vi "Annotation Holder.vi"(0 "Index":i32, 1 "Action":T2, 5 "Start time":timestamp, 7 "Annotation in":T1, 9 "End Time":timestamp, 11 "error in (no error)":errorcluster, 12 "Array of annotations in":T1[](array[typedef])) -> (4 "Index & Size Out":i32, 6 "Array of Indexes":i32[](array[numeric]), 8 "Annotation out":T1, 10 "Array Of annotations":T1[](array[typedef]), 15 "error out":errorcluster)   [LabVIEW 2011]
uses:
  Actin Annotatino Holder.ctl
  Annotation Message.ctl
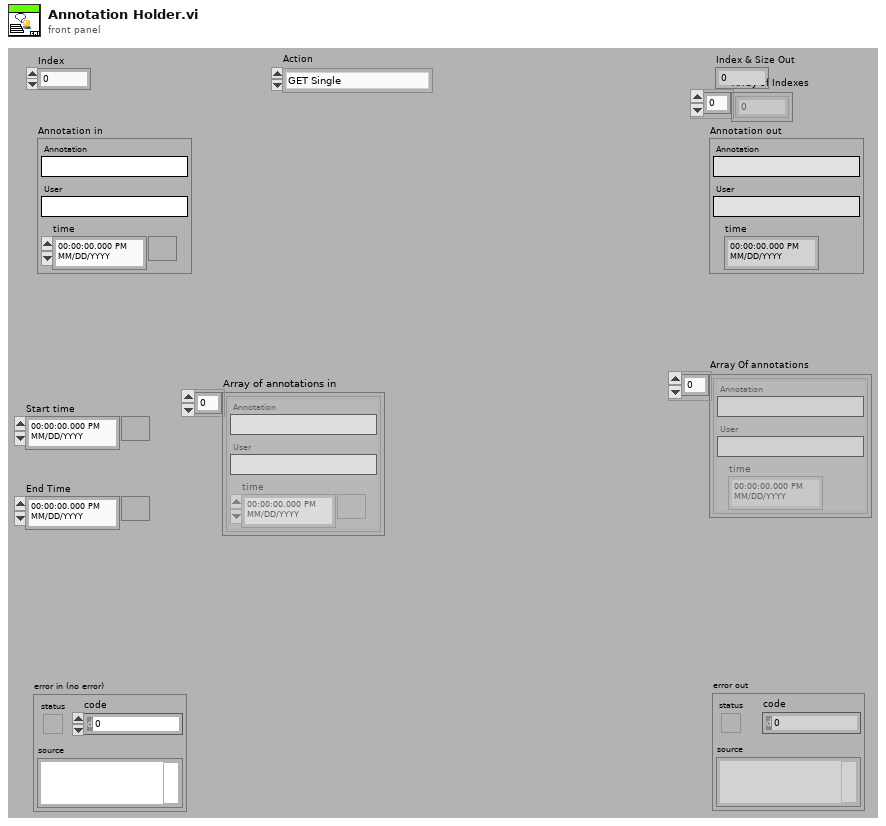
[diagram p1: front panel]
types:
  T1 = typedef "Annotation Message.ctl" = cluster{"Annotation":string, "User":string, "time":timestamp}
  T2 = typedef "Actin Annotatino Holder.ctl" = enum16{"GET Single", "GET All", "GET Time Period", "GET Index", "Get Size", "Add Single", "Replace Single", "Delete Single", "SET All"}
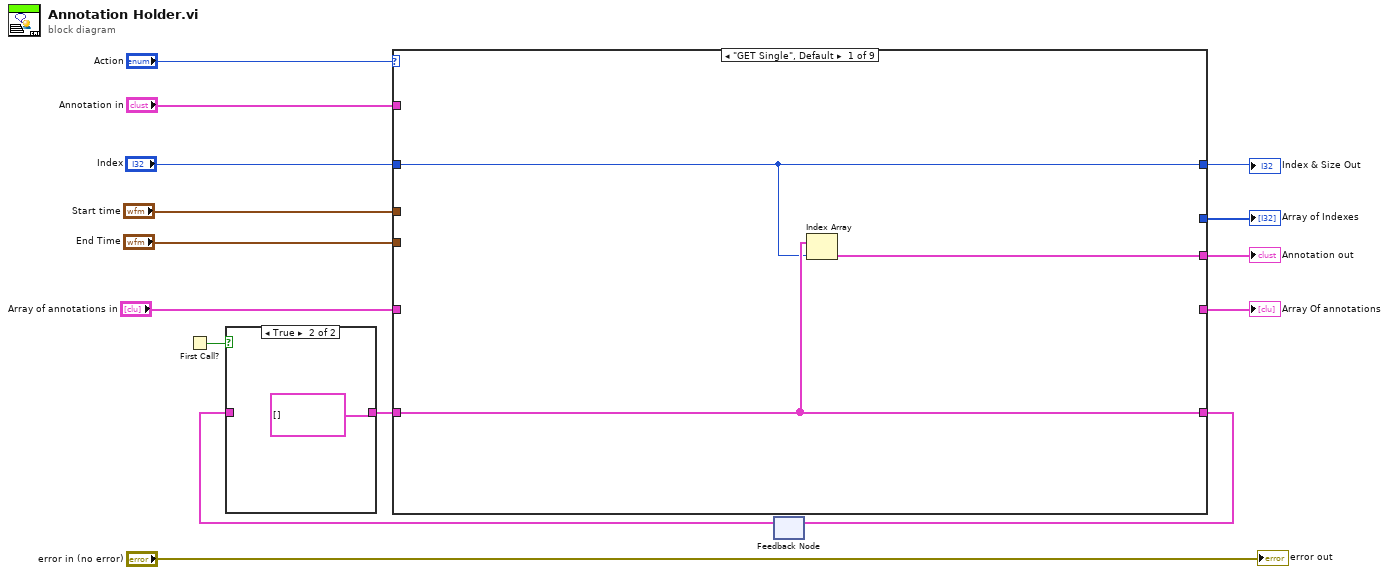
[diagram p0: block diagram]
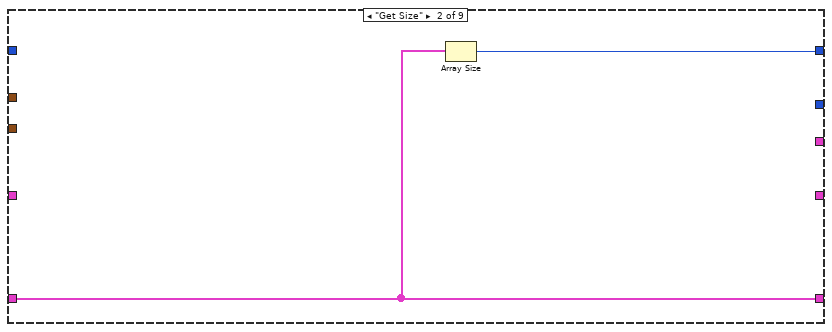
[diagram p3: hidden frame]
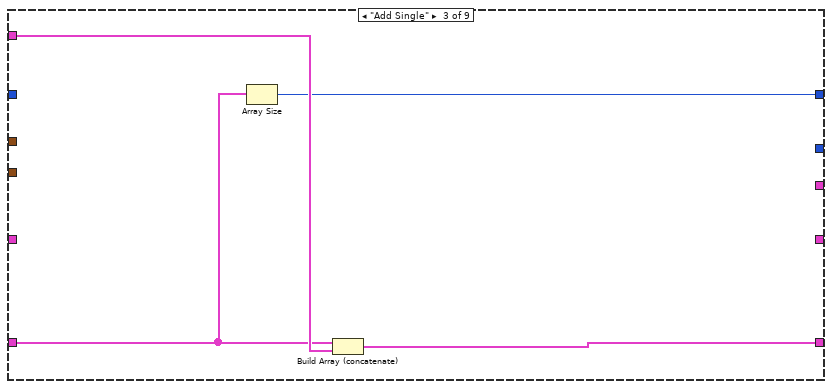
[diagram p4: hidden frame]
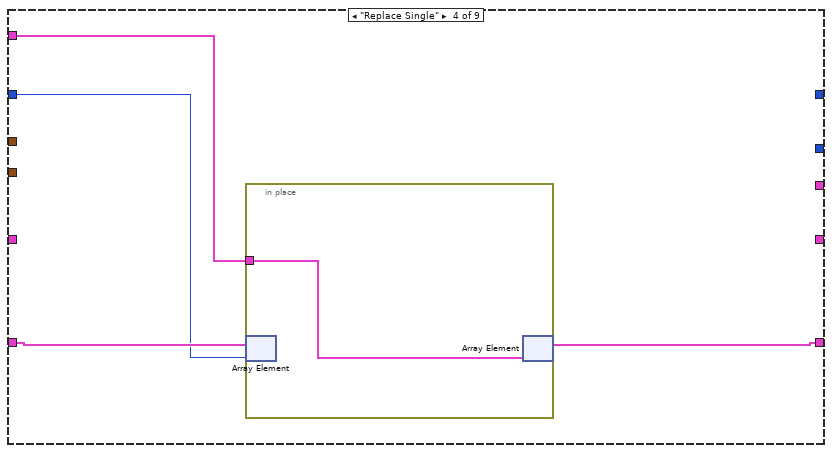
[diagram p5: hidden frame]
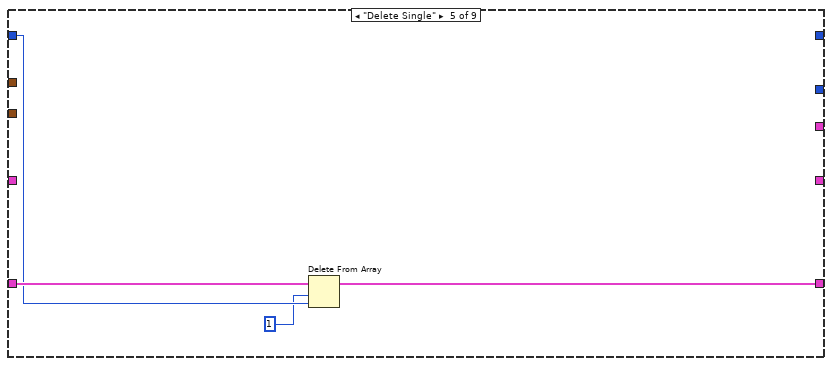
[diagram p6: hidden frame]
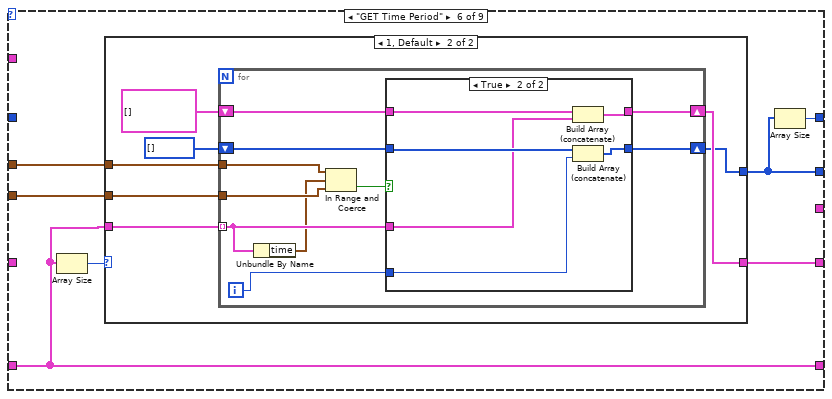
[diagram p7: hidden frame]
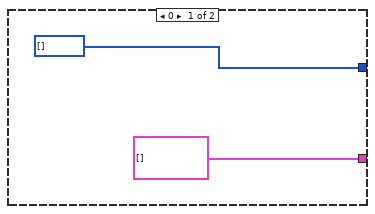
[diagram p8: hidden frame]
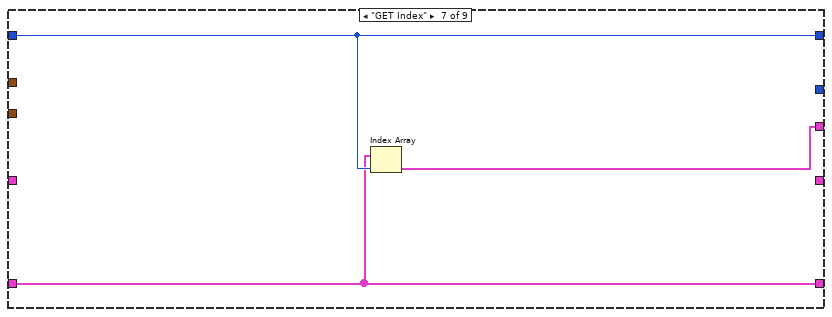
[diagram p10: hidden frame]
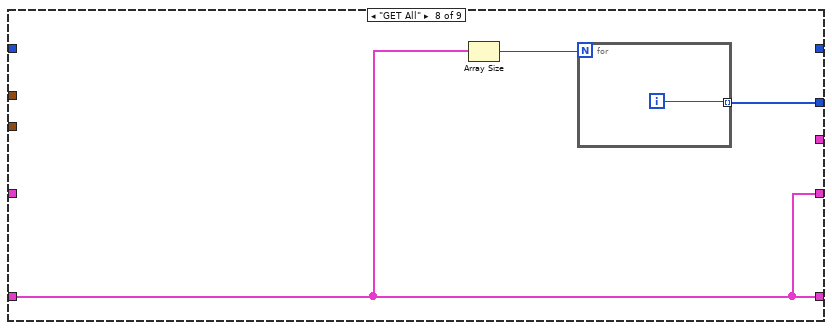
[diagram p11: hidden frame]
diagram:
  n1 = First Call?() -> (First Call?: T/F=w12:bool)
  n2 = feedback #1() -> (w13:T1[])  [unwired: 1 in]
  n3 = case shown="True" w12 {
    tunnel: w13 -> [w16 _]
    tunnel: [w16 T1[] []] -> w10
    frame False {
    }
    frame True {
    }
  }
  n4 = case shown="\"GET Single\", Default" "Action" {
    tunnel: [w20 w22 w26 w29 w34 w38 w71 w74 w77] -> w11
    tunnel: w10 -> [w20 w22 w24 w30 w35 w38 w71 w74 _]
    tunnel: "Annotation in" -> [_ _ w25 w27 _ _ _ _ _]
    tunnel: [_ _ _ _ _ w41 _ w74 _] -> w8
    tunnel: [_ _ _ _ _ w36 _ w75 _] -> w7
    tunnel: [w19 w21 w23 _ _ w37 w72 _ _] -> w6
    tunnel: "Index" -> [w19 _ _ w28 w33 _ w72 _ _]
    tunnel: [w18 _ _ _ _ _ w70 _ _] -> w4
    tunnel: "Start time" -> [_ _ _ _ _ w40 _ _ _]
    tunnel: "End Time" -> [_ _ _ _ _ w39 _ _ _]
    tunnel: "Array of annotations in" -> [_ _ _ _ _ _ _ _ w77]
    frame "GET Single", Default {
      n5 = Index Array(array=w20, index=w19) -> (element=w18:T1)
    }
    frame "Get Size" {
      n6 = Array Size(array=w22) -> (size(s)=w21:i32)
    }
    frame "Add Single" {
      n7 = Array Size(array=w24) -> (size(s)=w23:i32)
      n8 = Build Array (concatenate)(w24, w25) -> (w26:T1[])
    }
    frame "Replace Single" {
      n9 = in-place {
        in-place-border: w27 -> [w31]
        n10 = in-place-array #2(w30, w28) -> ()  [unwired: 1 out]
        n11 = in-place-array #2(w31) -> (w29:T1[])  [unwired: 1 out]
      }
    }
    frame "Delete Single" {
      n12 = Delete From Array(array=w35, length=1, index=w33) -> (array with subset deleted=w34:T1[])  [unwired: 1 out]
    }
    frame "GET Time Period" {
      n13 = Array Size(array=w38) -> (size(s)=w42:i32)
      n14 = case shown="1, Default" w42 {
        tunnel: [i32[] [] w45] -> w36
        tunnel: [T1[] [] w46] -> w41
        tunnel: w40 -> [_ w48]
        tunnel: w39 -> [_ w49]
        tunnel: w38 -> [_ w51]
        frame 0 {
        }
        frame 1, Default {
          n15 = for {
            tunnel: w51 -> [w61] mode=indexing
            shift-right: [w55] -> w46
            shift-left: T1[] [] -> [w56]
            tunnel: w49 -> [w59]
            tunnel: w48 -> [w60]
            shift-right: [w54] -> w45
            shift-left: i32[] [] -> [w53]
            i -> [w52]
            n16 = Unbundle By Name(w61) -> ("time"=w58:timestamp)
            n17 = In Range and Coerce(upper limit=w60, x=w58, lower limit=w59) -> (In Range?=w57:bool)  [unwired: 1 out]
            n18 = case shown="True" w57 {
              tunnel: w61 -> [_ w66]
              tunnel: w56 -> [w63 w65]
              tunnel: [w63 w64] -> w55
              tunnel: [w62 w68] -> w54
              tunnel: w53 -> [w62 w69]
              tunnel: w52 -> [_ w67]
              frame False {
              }
              frame True {
                n19 = Build Array (concatenate)(w65, w66) -> (w64:T1[])
                n20 = Build Array (concatenate)(w69, w67) -> (w68:i32[])
              }
            }
          }
        }
      }
      n21 = Array Size(array=w36) -> (size(s)=w37:i32)
    }
    frame "GET Index" {
      n22 = Index Array(array=w71, index=w72) -> (element=w70:T1)
    }
    frame "GET All" {
      n23 = Array Size(array=w74) -> (size(s)=w73:i32)
      n24 = for {
        N: w73 -> [_]
        tunnel: [w76] -> w75 mode=indexing
        i -> [w76]
      }
    }
    frame "SET All" {
    }
  }
  "Annotation out" <- w4
  "Array Of annotations" <- w8
  "Array of Indexes" <- w7
  "Index & Size Out" <- w6
  n25 = feedback-in #1(w11) -> ()
  "error out" <- "error in (no error)"
